vi "valueFromText.vi"(8 "Error In":errorcluster, 10 "text":string, 11 "QDoubleSpinBox In":refnum<class "QDoubleSpinBox.lvclass">) -> (0 "Error Out":errorcluster, 2 "Value":dbl, 3 "QDoubleSpinBox Out":refnum<class "QDoubleSpinBox.lvclass">)   [LabVIEW 2014, in "QDoubleSpinBox.lvclass"]
doc: "LabVIEW-specific documentation is not yet available. See <b>https://doc.qt.io/qt-5/qdoublespinbox.html#valueFromText</b>"
uses:
  QDoubleSpinBox.lvclass
  LQ Core/LQIdentity/LQIdentity.lvclass/LQIdentity.ctl
  LQ Core/LQ Core.lvlib
  LQ Core/LQIdentity/LQIdentity.lvclass
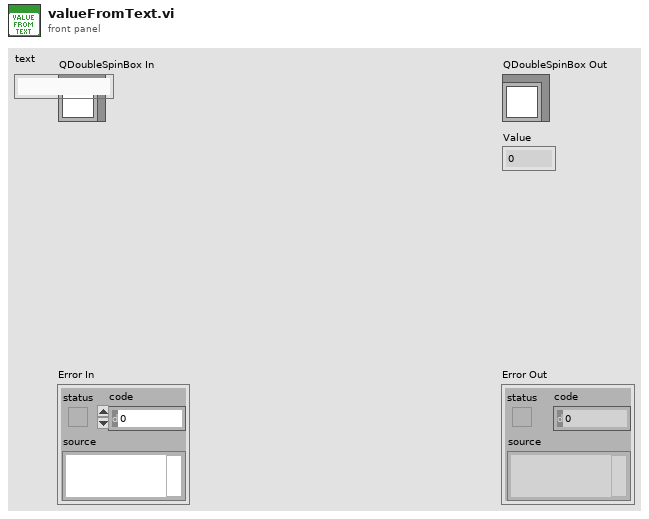
[diagram p1: front panel]
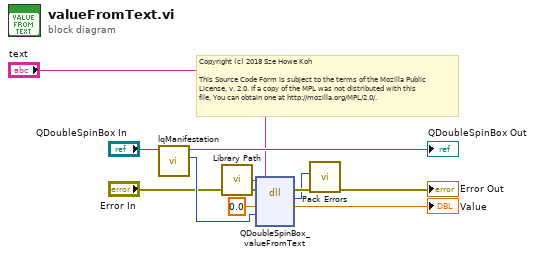
[diagram p0: block diagram]
diagram:
  # "Copyright (c) 2018 Sze Howe Koh\n\nThis Source Code Form is subject to the terms of the Mozilla Public\nLicense, v. 2.0. If a copy of the MPL was not distributed with this\nfile, You can obtain one at http://mozilla.org/MPL/2.0/."
  n1 = call "lqManifestation.vi"("LQIdentity in"="QDoubleSpinBox In") -> ("Manifestation"=w6:u64, "LQIdentity out"=→"QDoubleSpinBox Out":refnum<class "QDoubleSpinBox.lvclass">)  [unwired: 9 in]
  n2 = call "Library Path.vi"() -> ("Library Path"=w7:path)
  n3 = dll-call lib="?" fn="QDoubleSpinBox_valueFromText"(path in=w7, error in="Error In", "_retVal"=0.0 ("retVal"), "_instance"=w6, "text"="text") -> (error out=w4:errorcluster, w2:i32, "_retVal"=→"Value":dbl)  [unwired: 3 in, 1 out]
  n4 = call "Pack Errors.vi"("Error In"=w4, "Error Code"=w2) -> ("Error Out"=→"Error Out":errorcluster)  [unwired: 9 in]
